vi "CalcCRC.vi"(8 "error in (no error)":errorcluster, 10 "TextIn":string, 11 "object in":refnum<class "CRC16.lvclass">) -> (0 "error out":errorcluster, 2 "CrcOut":string, 3 "object out":refnum<class "CRC16.lvclass">)   [LabVIEW 2020, in "CRC Implementations.lvlib" / "CRC16.lvclass"]
uses:
  CRC16.lvclass
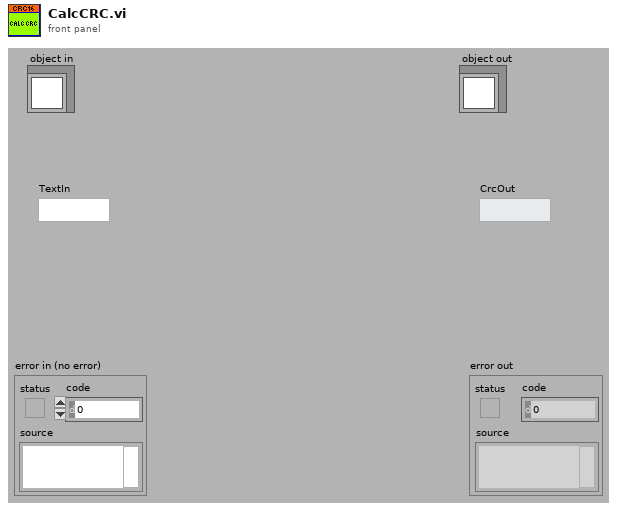
[diagram p1: front panel]
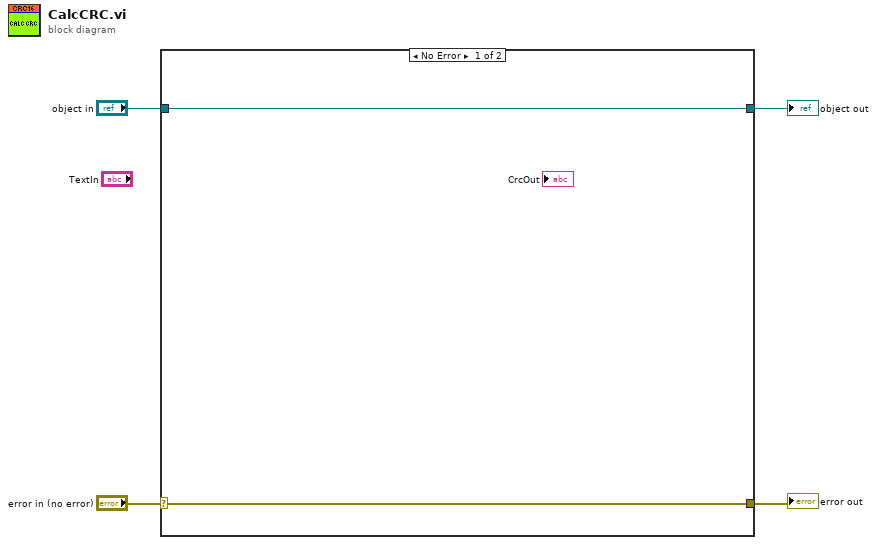
[diagram p0: block diagram]
diagram:
  n1 = case shown="No Error" "error in (no error)" {
    selector: "error in (no error)" -> [w5 w8]
    tunnel: [w5 w8] -> w3
    tunnel: [w6 w7] -> w1
    tunnel: "object in" -> [w6 w7]
    frame No Error {
    }
    frame Error {
    }
  }
  "error out" <- w3
  "object out" <- w1
